vi "get_path_sfx.vi"(8 "error in (no error)":errorcluster) -> (0 "error out":errorcluster, 3 "sfx":path)   [LabVIEW 2015, in "lv-bin-7zip.lvlib"]
uses:
  lv-bin-7zip.lvlib
  public/_controls/error.ctl
  _controls/files.ctl
  <userlib>/antonio-alexander/lv-bin/public/api/v1/v1.lvlib
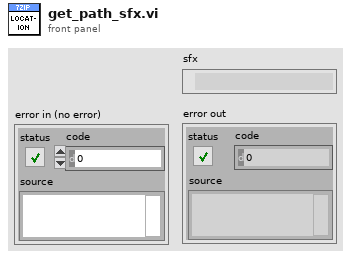
[diagram p1: front panel]
types:
  T1 = typedef "lv-bin-7zip.lvlib/files.ctl" = enum16{"<7z_file>", "7z.dll", "7z.exe", "7z.sfx", "7zCon.sfx", "7zFM. exe", "7zG.exe"}
  T2 = typedef "lv-bin-7zip.lvlib/error.ctl" = enum16{"<error>", "exe_x86_missing", "exe_x64_missing", "7za_x86_missing", "7za_x64_missing", "7zxa_x86_missing", "7zxa_x64_missing", "7zS.sfx_missing", "7z.exe_missing"}
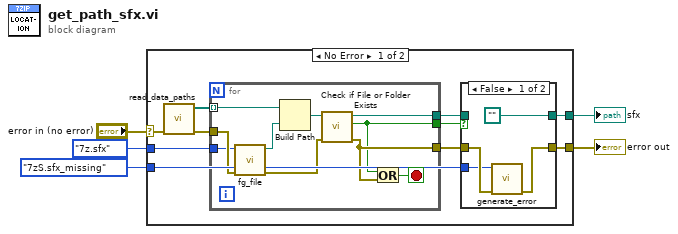
[diagram p0: block diagram]
diagram:
  n1 = case shown="No Error" "error in (no error)" {
    selector: "error in (no error)" -> [w15 w32]
    tunnel: [w8 w32] -> w1
    tunnel: [w10 _] -> w2
    tunnel: error."7zS.sfx_missing" ("error") -> [w7 _]
    tunnel: files."7z.sfx" ("files") -> [w6 _]
    frame No Error {
      n2 = call <userlib>:"read_data_paths.vi"("error in (no error)"=w15) -> ("error out"=w14:errorcluster, "path [] out"=w13:path[])  [unwired: 9 in]
      n3 = for {
        tunnel: w13 -> [w24] mode=indexing
        tunnel: [w25] -> w12
        tunnel: [w21] -> w11
        tunnel: w14 -> [w18]
        tunnel: [w23] -> w9
        tunnel: w6 -> [w16]
        stop <- w22 stop-if-true
        n4 = call "fg_file.vi"("error in (no error)"=w18, "files"=w16) -> ("error out"=w17:errorcluster, "file"=w19:path)  [unwired: 8 in]
        n5 = Build Path(base path=w24, name or relative path=w19) -> (appended path=w20:path)
        n6 = call <vilib>:"Check if File or Folder Exists.vi"("error in (no error)"=w17, "path"=w20) -> ("error out"=w23:errorcluster, "file or folder exists?"=w21:bool, "dup path"=w25:path)  [unwired: 7 in]
        n7 = Or(x=w21, y=w23) -> (x .or. y?=w22:bool)
      }
      n8 = case shown="False" w11 {
        tunnel: w12 -> [_ w31]
        tunnel: [path "" w31] -> w10
        tunnel: w9 -> [w29 w30]
        tunnel: [w28 w30] -> w8
        tunnel: w7 -> [w26 _]
        frame False {
          n9 = call "generate_error.vi"("error in (no error)"=w29, "error"=w26) -> ("error out"=w28:errorcluster)  [unwired: 9 in]
        }
        frame True {
        }
      }
    }
    frame Error {
    }
  }
  "error out" <- w1
  "sfx" <- w2
